vi "Write Job.vi"(10 "Job.lvclass":refnum<class "Job.lvclass">, 11 "Jobber in":refnum<class "Jobber.lvclass">) -> (3 "Jobber out":refnum<class "Jobber.lvclass">)   [LabVIEW 2014, in "Jobber.lvlib" / "Jobber.lvclass"]
uses:
  Jobber.lvclass
  Classes/Job/Job.lvclass
  Jobber.lvclass/Jobber.ctl
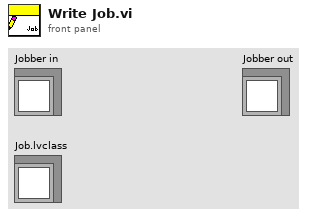
[diagram p1: front panel]
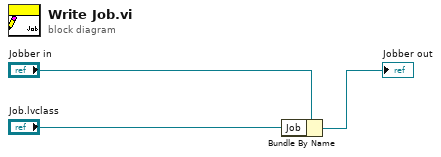
[diagram p0: block diagram]
diagram:
  n1 = Bundle By Name(cluster="Jobber in", "Job"="Job.lvclass") -> (→"Jobber out":refnum<class "Jobber.lvclass">)
